vi "PFE_INITIAL (SubVI).vi"(10 "Cluster":T1, 11 "CONNECT WITH PFEIFFER":bool) -> (0 "error out":errorcluster, 1 "Gauge out":string[](array[string]), 2 "Serial Number":string, 3 "Referenz out":refnum<visa-resource-name>, 5 "Device Type":string)   [LabVIEW 2020]
uses:
  Desktop/eTPC/subVIs for MKS/INITIALIZATION PFEIFFER.ctl
  <instrlib>/PV ActiveLine/PV ActiveLine.lvlib
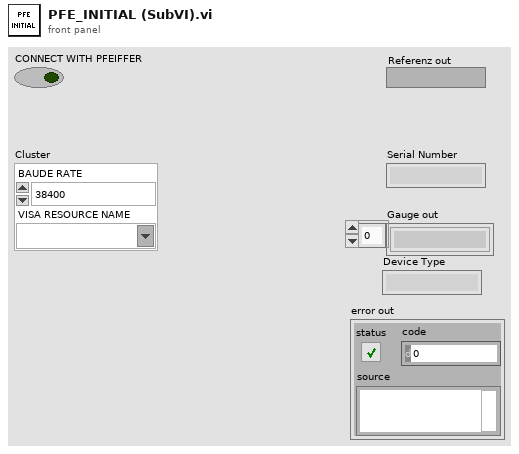
[diagram p1: front panel]
types:
  T1 = typedef "INITIALIZATION PFEIFFER.ctl" = cluster{"BAUDE RATE":enum32{"38400", "19200", "9600", "4800"}, "VISA RESOURCE NAME":refnum<visa-resource-name>}
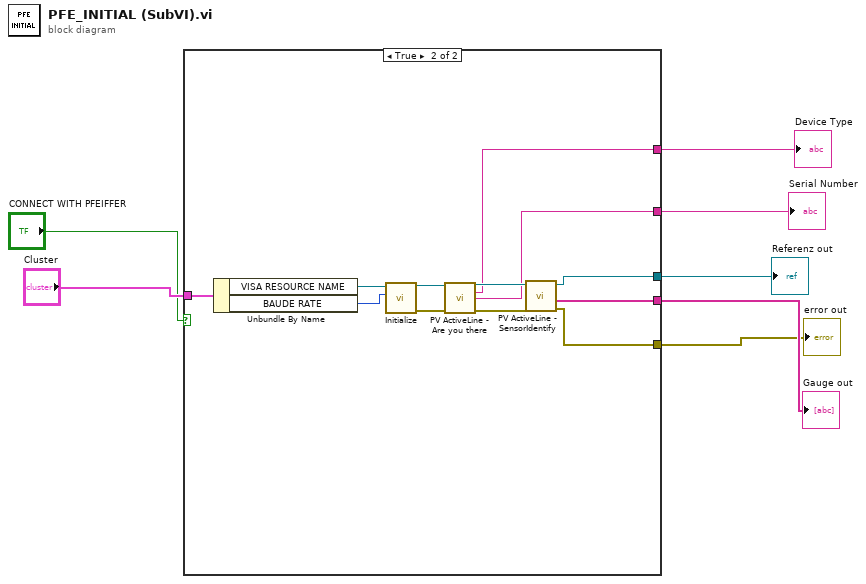
[diagram p0: block diagram]
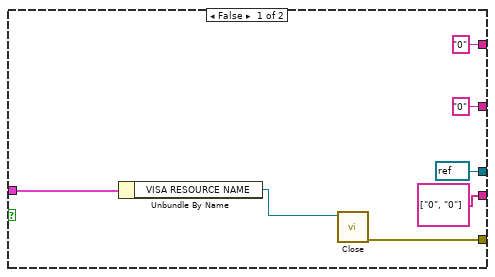
[diagram p2: hidden frame]
diagram:
  n1 = case shown="True" "CONNECT WITH PFEIFFER" {
    tunnel: [w14 w19] -> w3
    tunnel: "Cluster" -> [w13 w26]
    tunnel: ["0" ("Serial Number") w18] -> w5
    tunnel: ["0" ("Device Type") w17] -> w6
    tunnel: [string[] ["0", "0"] ("Gauge out") w16] -> w7
    tunnel: [refnum<visa-resource-name> refnum ("Referenz out") w15] -> w1
    frame False {
      n2 = Unbundle By Name(w13) -> ("VISA RESOURCE NAME"=w12:refnum<visa-resource-name>)
      n3 = call <instrlib>:"Close.vi"("VISA resource name"=w12) -> ("error out"=w14:errorcluster)  [unwired: 10 in]
    }
    frame True {
      n4 = Unbundle By Name(w26) -> ("VISA RESOURCE NAME"=w25:refnum<visa-resource-name>, "BAUDE RATE"=w24:enum32{"38400", "19200", "9600", "4800"})
      n5 = call <instrlib>:"Initialize.vi"("Baud Rate"=w24, "input refnum"=w25) -> ("Cluster (Ausgang)"=w22:errorcluster, "Referenz out"=w23:refnum<visa-resource-name>)  [unwired: 8 in]
      n6 = call <instrlib>:"PV ActiveLine - Are you there.vi"("Referenz in"=w23, "Fehler (Eingang)"=w22) -> ("Referenz out"=w21:refnum<visa-resource-name>, "Device Type"=w17:string, "Serial Number"=w18:string, "Cluster (Ausgang)"=w20:errorcluster)  [unwired: 7 in, 3 out]
      n7 = call <instrlib>:"PV ActiveLine - SensorIdentify.vi"("Fehler (Eingang)"=w20, "Referenz in"=w21) -> ("Cluster (Ausgang)"=w19:errorcluster, "Gauge out"=w16:string[], "Referenz out"=w15:refnum<visa-resource-name>)  [unwired: 7 in]
    }
  }
  "Gauge out" <- w7
  "Device Type" <- w6
  "Serial Number" <- w5
  "error out" <- w3
  "Referenz out" <- w1
